vi "toXml.vi"(8 "error in (no error)":errorcluster, 11 "ScriptEvent in":refnum<class "ScriptEvent.lvclass">) -> (0 "error out":errorcluster, 2 "scriptEventXML":refnum<class "xmlNode.lvclass">, 3 "ScriptEvent out":refnum<class "ScriptEvent.lvclass">)   [LabVIEW 2011, in "Tools.lvlib" / "Scripting.lvlib" / "ScriptEvent.lvclass"]
uses:
  ScriptEvent.lvclass
  xmlNode/xmlNode.lvclass
  ScriptEvent.lvclass/ScriptEvent.ctl
  DatabaseHelpers/Database Objects/Channel/Channel.lvclass
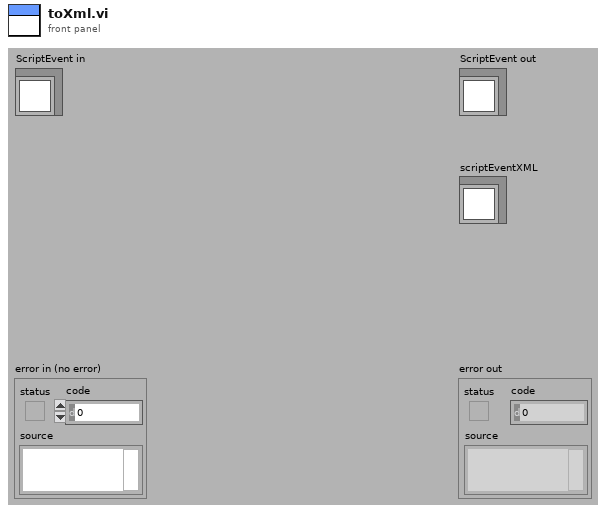
[diagram p1: front panel]
types:
  T1 = cluster{"attributeName":string, "channel_name":string}
  T2 = cluster{"attributeName":string, "channel_name":string}[]
  T3 = cluster{"parameter_name":string, "parameter_value":string, "type":enum16{"time", "time_difference", "value", "frequency", "phase", "ramp_time", "value_step", "time_step", "number_of_steps", "start_value", "end_value", "start_freq", "start_amp", "start_phase", "end_freq", "end_amp", "end_phase"}}[]
  T4 = enum16{"time", "time_difference", "value", "frequency", "phase", "ramp_time", "value_step", "time_step", "number_of_steps", "start_value", "end_value", "start_freq", "start_amp", "start_phase", "end_freq", "end_amp", "end_phase"}
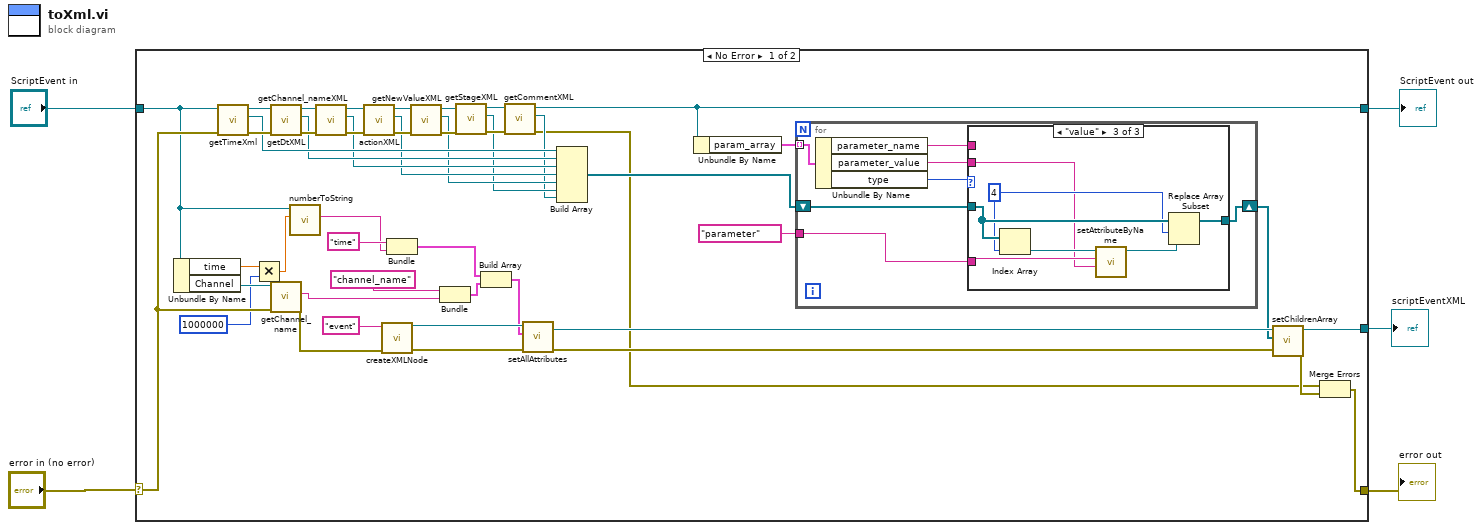
[diagram p0: block diagram]
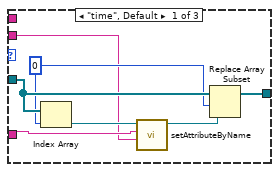
[diagram p2: hidden frame]
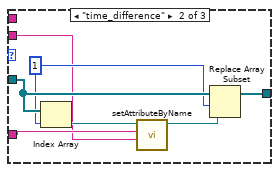
[diagram p3: hidden frame]
diagram:
  n1 = case shown="No Error" "error in (no error)" {
    selector: "error in (no error)" -> [w37 w82]
    tunnel: [w28 w82] -> w4
    tunnel: [w12 w81] -> w2
    tunnel: "ScriptEvent in" -> [w13 w81]
    tunnel: [w8 _] -> w1
    frame No Error {
      n2 = Unbundle By Name(w13) -> ("time"=w17:dbl, "Channel"=w51:refnum<class "Channel.lvclass">)
      n3 = call "getTimeXml.vi"("error in (no error)"=w37, "ScriptEvent in"=w13) -> ("error out"=w49:errorcluster, "timeXML"=w36:refnum<class "xmlNode.lvclass">, "ScriptEvent out"=w43:refnum<class "ScriptEvent.lvclass">)  [unwired: 7 in]
      n4 = Multiply(x=w17, y=1000000) -> (x*y=w15:dbl)
      n5 = call "getDtXML.vi"("error in (no error)"=w49, "ScriptEvent in"=w43) -> ("error out"=w48:errorcluster, "dtXML"=w35:refnum<class "xmlNode.lvclass">, "ScriptEvent out"=w42:refnum<class "ScriptEvent.lvclass">)  [unwired: 7 in]
      n6 = call "getChannel_name.vi"("error in (no error)"=w37, "Channel.lvclass in"=w51) -> ("error out"=w50:errorcluster, "channel_name"=w25:string)  [unwired: 7 in, 1 out]
      n7 = call "numberToString.vi"("Numeric"=w15, "ScriptEvent in"=w13) -> ("String"=w14:string)  [unwired: 7 in, 2 out]
      n8 = call "getChannel_nameXML.vi"("error in (no error)"=w48, "ScriptEvent in"=w42) -> ("error out"=w47:errorcluster, "channel_nameXML"=w34:refnum<class "xmlNode.lvclass">, "ScriptEvent out"=w41:refnum<class "ScriptEvent.lvclass">)  [unwired: 7 in]
      n9 = call "actionXML.vi"("error in (no error)"=w47, "ScriptEvent in"=w41) -> ("error out"=w46:errorcluster, "actionXml"=w33:refnum<class "xmlNode.lvclass">, "ScriptEvent out"=w40:refnum<class "ScriptEvent.lvclass">)  [unwired: 7 in]
      n10 = call "createXMLNode.vi"("error in (no error)"=w50, "name"="event") -> ("error out"=w20:errorcluster, "xmlNode out"=w24:refnum<class "xmlNode.lvclass">)  [unwired: 8 in]
      n11 = Bundle("attributeName"="time", "String"=w14) -> (w23:cluster{"attributeName":string, "String":string})  [unwired: 1 in]
      n12 = call-dynamic "getNewValueXML.vi"("error in (no error)"=w46, "ScriptEvent in"=w40) -> ("error out"=w45:errorcluster, "newValueXML"=w32:refnum<class "xmlNode.lvclass">, "ScriptEvent out"=w39:refnum<class "ScriptEvent.lvclass">)  [unwired: 7 in]
      n13 = Bundle("attributeName"="channel_name", "channel_name"=w25) -> (w22:T1)  [unwired: 1 in]
      n14 = call "getStageXML.vi"("error in (no error)"=w45, "ScriptEvent in"=w39) -> ("error out"=w44:errorcluster, "stageXML"=w31:refnum<class "xmlNode.lvclass">, "ScriptEvent out"=w38:refnum<class "ScriptEvent.lvclass">)  [unwired: 7 in]
      n15 = Build Array(w23, w22) -> (w21:T2)
      n16 = call "getCommentXML.vi"("error in (no error)"=w44, "ScriptEvent in"=w38) -> ("error out"=w7:errorcluster, "commentXML"=w30:refnum<class "xmlNode.lvclass">, "ScriptEvent out"=w12:refnum<class "ScriptEvent.lvclass">)  [unwired: 7 in]
      n17 = call-dynamic "setAllAttributes.vi"("error in (no error)"=w20, "attributes"=w21, "xmlNode in"=w24) -> ("error out"=w19:errorcluster, "xmlNode out"=w18:refnum<class "xmlNode.lvclass">)  [unwired: 7 in]
      n18 = Build Array(w36, w35, w34, w33, w32, w31, w30) -> (w10:refnum<class "xmlNode.lvclass">[])
      n19 = Unbundle By Name(w12) -> ("param_array"=w11:T3)
      n20 = for {
        tunnel: w11 -> [w59] mode=indexing
        shift-right: [w54] -> w9
        shift-left: w10 -> [w57]
        tunnel: "parameter" -> [w53]
        n21 = Unbundle By Name(w59) -> ("parameter_name"=w56:string, "parameter_value"=w55:string, "type"=w58:T4)
        n22 = case shown="\"value\"" w58 {
          tunnel: w57 -> [w64 w71 w78]
          tunnel: w56 -> [_ _ _]
          tunnel: w55 -> [w60 w67 w74]
          tunnel: [w62 w69 w76] -> w54
          tunnel: w53 -> [w61 w68 w75]
          frame "time", Default {
            w63 = 0
            n23 = Index Array(array=w64, index=w63) -> (element=w66:refnum<class "xmlNode.lvclass">)
            n24 = call-dynamic "setAttributeByName.vi"("attributeValue"=w60, "attributeName"=w61, "xmlNode in"=w66) -> ("xmlNode out"=w65:refnum<class "xmlNode.lvclass">)  [unwired: 7 in, 1 out]
            n25 = Replace Array Subset(array=w64, new element=w65, index=w63) -> (w62:refnum<class "xmlNode.lvclass">[])
          }
          frame "time_difference" {
            w70 = 1
            n26 = Index Array(array=w71, index=w70) -> (element=w73:refnum<class "xmlNode.lvclass">)
            n27 = call-dynamic "setAttributeByName.vi"("attributeValue"=w67, "attributeName"=w68, "xmlNode in"=w73) -> ("xmlNode out"=w72:refnum<class "xmlNode.lvclass">)  [unwired: 7 in, 1 out]
            n28 = Replace Array Subset(array=w71, new element=w72, index=w70) -> (w69:refnum<class "xmlNode.lvclass">[])
          }
          frame "value" {
            w77 = 4
            n29 = Index Array(array=w78, index=w77) -> (element=w80:refnum<class "xmlNode.lvclass">)
            n30 = call-dynamic "setAttributeByName.vi"("attributeValue"=w74, "attributeName"=w75, "xmlNode in"=w80) -> ("xmlNode out"=w79:refnum<class "xmlNode.lvclass">)  [unwired: 7 in, 1 out]
            n31 = Replace Array Subset(array=w78, new element=w79, index=w77) -> (w76:refnum<class "xmlNode.lvclass">[])
          }
        }
      }
      n32 = call-dynamic "setChildrenArray.vi"("error in (no error)"=w19, "Children"=w9, "xmlNode.lvclass in"=w18) -> ("error out"=w29:errorcluster, "xmlNode.lvclass out"=w8:refnum<class "xmlNode.lvclass">)  [unwired: 7 in]
      n33 = Merge Errors(w7, w29) -> (w28:errorcluster)
    }
    frame Error {
    }
  }
  "error out" <- w4
  "ScriptEvent out" <- w2
  "scriptEventXML" <- w1
